vi "5000error.vi"(1 "String":string) -> (0 "x UND y?":bool)   [LabVIEW 2017]
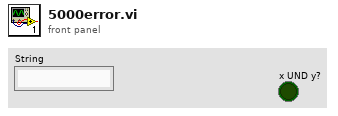
[diagram p1: front panel]
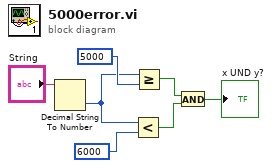
[diagram p0: block diagram]
diagram:
  n1 = Decimal String To Number(string="String") -> (number=w1:i32)  [unwired: 2 in, 1 out]
  n2 = Less?(x=w1, y=6000) -> (x < y?=w6:bool)
  n3 = Greater Or Equal?(x=w1, y=5000) -> (x >= y?=w7:bool)
  n4 = And(x=w7, y=w6) -> (x .and. y?=→"x UND y?":bool)
